vi "FGVTimer.vi"(8 "error in":errorcluster, 11 "Reset":bool) -> (0 "error out":errorcluster, 2 "Elapsed?":bool, 3 "Time Elapsed":dbl)   [LabVIEW 2019]
doc: "Timer semplice che si basa su un numero random come limite di tempo massimo"
uses:
  <vilib>/numeric/Random Number (Range) DBL.vi
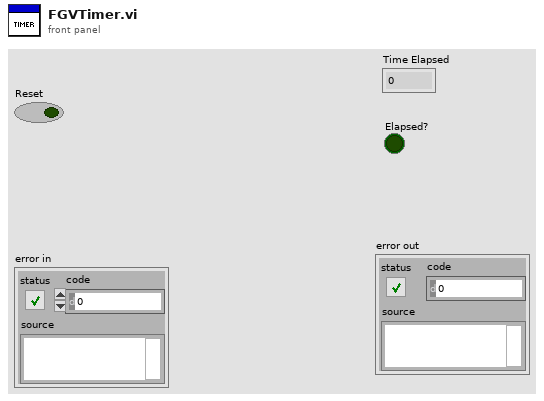
[diagram p1: front panel]
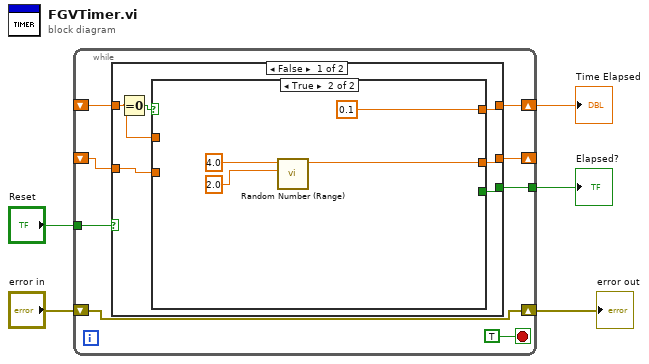
[diagram p0: block diagram]
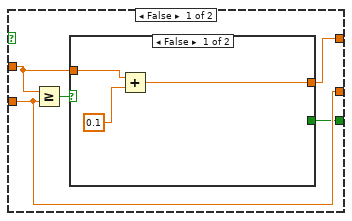
[diagram p2: hidden frame]
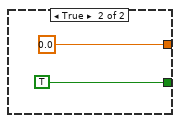
[diagram p3: hidden frame]
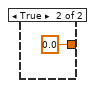
[diagram p4: hidden frame]
diagram:
  n1 = while {
    shift-right: [w12] -> w5
    shift-left: _ -> [w11]
    shift-right: [w10] -> _
    shift-left: _ -> [w9]
    tunnel: [w8] -> w4
    shift-right: [w7] -> w2
    shift-left: "error in" -> [w7]
    tunnel: "Reset" -> [w6]
    stop <- TRUE stop-if-true
    n2 = case shown="False" w6 {
      tunnel: [w19 0.0] -> w12
      tunnel: w11 -> [w17 _]
      tunnel: [w16 _] -> w10
      tunnel: w9 -> [w15 _]
      tunnel: [w14 _] -> w8
      frame False {
        n3 = Equal To 0?(x=w17) -> (x = 0?=w18:bool)
        n4 = case shown="True" w18 {
          tunnel: [w22 0.1] -> w19
          tunnel: w17 -> [w23 _]
          tunnel: [w21 w30] -> w16
          tunnel: w15 -> [w21 _]
          tunnel: [w20 _] -> w14
          frame False {
            n5 = Greater Or Equal?(x=w23, y=w21) -> (x >= y?=w24:bool)
            n6 = case shown="False" w24 {
              tunnel: w23 -> [w27 _]
              tunnel: [w25 0.0] -> w22
              tunnel: [_ TRUE] -> w20
              frame False {
                n7 = Add(x=w27, y=0.1) -> (x+y=w25:dbl)
              }
              frame True {
              }
            }
          }
          frame True {
            n8 = call-poly <vilib>:"Random Number (Range).vi"("lower bound (0)"=2.0, "upper bound (100)"=4.0) -> ("number"=w30:dbl)  [unwired: 9 in]
          }
        }
      }
      frame True {
      }
    }
  }
  "Time Elapsed" <- w5
  "Elapsed?" <- w4
  "error out" <- w2
